vi "Test Saturated Sin Multi.vi"() -> ()   [LabVIEW 2017]
uses:
  <vilib>/Utility/file.llb/Read Delimited Spreadsheet (DBL).vi
panel:
  out "min value":dbl
  out "max value":dbl
  out "Range":dbl
  out "Error":bool
  out "Mean Current 2":dbl[](array[numeric]) format="%#.3g"
  out "Waveform Graph 3":dbl[][](graph)
  in  "Next":bool
  out "Currents":dbl[](array[numeric])
  out "mean":dbl format="%0.2f"
  out "String":string
  in  "Path":path
  out "Errors":dbl[](array[numeric])
  out "Mean Current":dbl[](array[numeric]) format="%#.3g"
  out "Waveform Graph":dbl[][](graph)
  out "all rows":dbl[][](array[numeric])
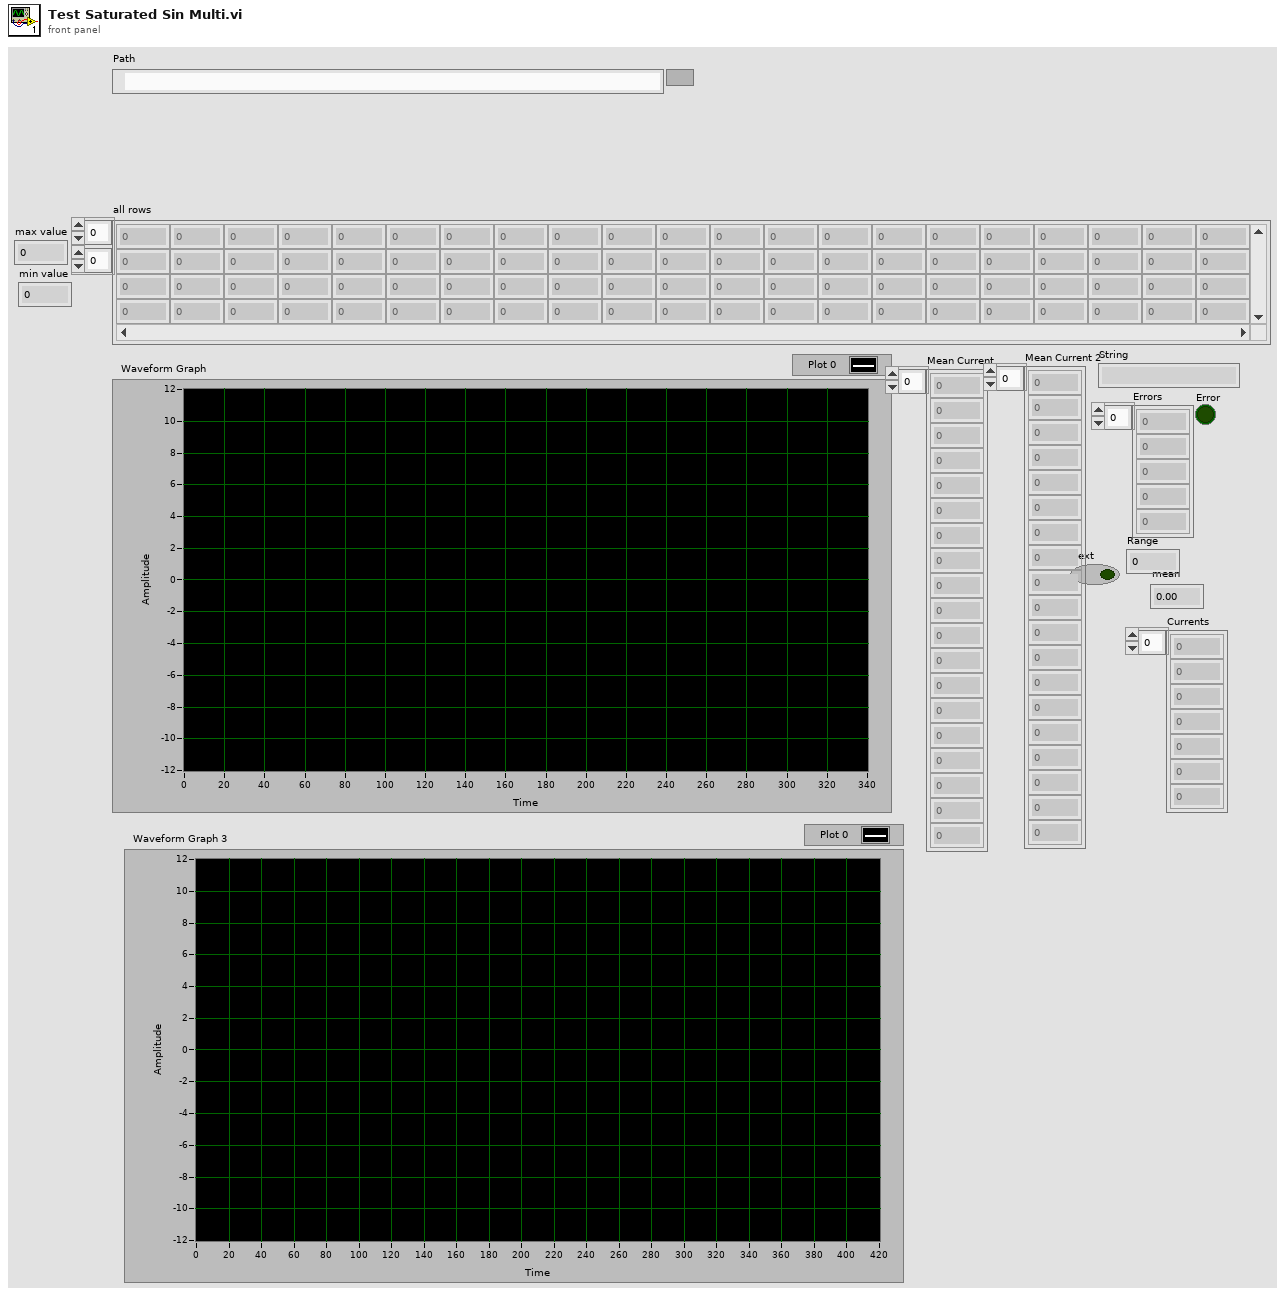
[diagram p1: front panel]
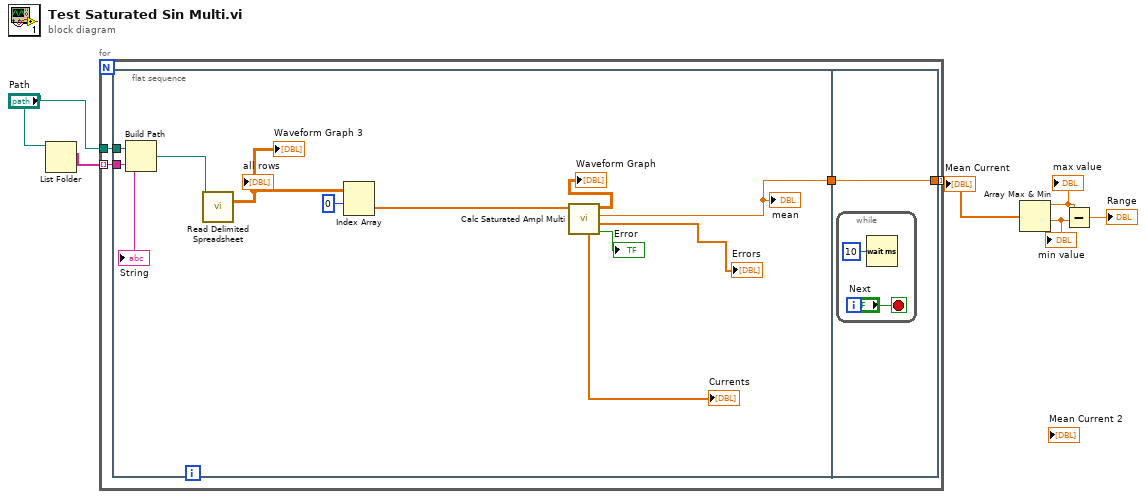
[diagram p0: block diagram]
diagram:
  n1 = List Folder(path="Path") -> (filenames=w5:string[])  [unwired: 3 in, 3 out]
  n2 = for {
    tunnel: "Path" -> [w10]
    tunnel: w5 -> [w9] mode=indexing
    tunnel: [w8] -> w1 mode=indexing
    n3 = flat-sequence {
      tunnel: w10 -> [w19]
      tunnel: w9 -> [w18]
      tunnel: [w16] -> w7
      tunnel: [w22] -> w8
      tunnel: w7 -> [w22]
      frame #0 {
        n4 = Build Path(base path=w19, name or relative path=w18) -> (appended path=w17:path)
        n5 = call-poly <vilib>:"Read Delimited Spreadsheet.vi"("file path (dialog if empty)"=w17) -> ("all rows"=w15:dbl[][])  [unwired: 9 in, 5 out]
        "all rows" <- w15
        "Waveform Graph 3" <- w15
        n6 = Index Array(array=w15, index (row)=0) -> (element=w20:dbl[])  [unwired: 1 in]
        n7 = call "Calc Saturated Ampl Multi.vi"("Data"=w20) -> ("Error"=→"Error":bool, "Errors"=→"Errors":dbl[], "mean"=w16:dbl, "Waveform Graph"=→"Waveform Graph":dbl[][], "Currents"=→"Currents":dbl[])  [unwired: 6 in]
        "mean" <- w16
        "String" <- w18
      }
      frame #1 {
        n8 = while {
          stop <- "Next" stop-if-true
          n9 = Wait (ms)(milliseconds to wait=u32 10) -> ()  [unwired: 1 out]
        }
      }
    }
  }
  "Mean Current" <- w1
  n10 = Array Max & Min(array=w1) -> (max value=w2:dbl, min value=w3:dbl)  [unwired: 2 out]
  "max value" <- w2
  "min value" <- w3
  n11 = Subtract(x=w2, y=w3) -> (x-y=→"Range":dbl)
